vi "Node - Writer.vi"(8 "error in (no error)":errorcluster, 11 "Node Data In":T1) -> (0 "error out":errorcluster, 3 "Node Data Out":T1)   [LabVIEW 2016, in "PXImc Router.lvlib"]
uses:
  PXImc Router.lvlib
  Controls/Node Data.ctl
  <vilib>/NI Veristand/VeriStand Data/Byte Buffer/Byte Buffer.lvclass
  Controls/Node/Node - PXImc Parameters.ctl
  Controls/Node/Transfer Data.ctl
  Controls/Node/Node Ch Properties.ctl
  Controls/Data Type.ctl
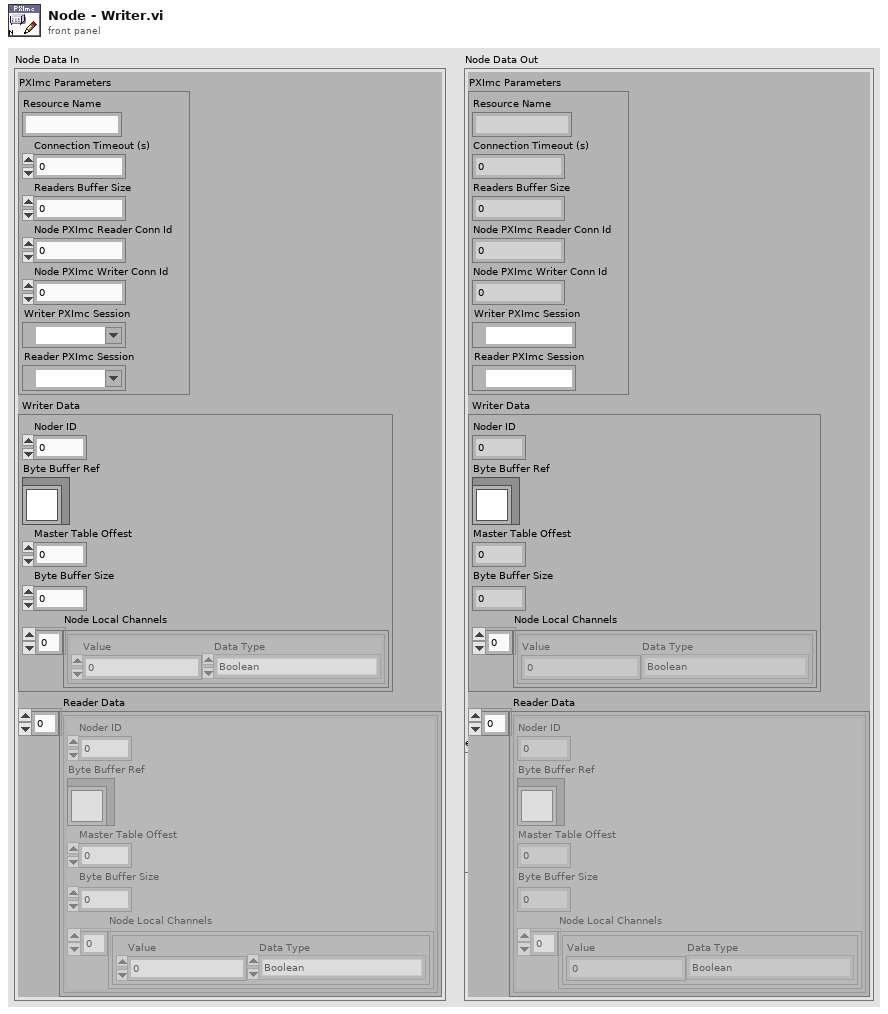
[diagram p1: front panel]
types:
  T1 = typedef "PXImc Router.lvlib/Node Data.ctl" = cluster{"PXImc Parameters":T2, "Writer Data":T3, "Reader Data":T3[]}
  T2 = typedef "PXImc Router.lvlib/Node - PXImc Parameters.ctl" = cluster{"Resource Name":string, "Connection Timeout (s)":dbl, "Readers Buffer Size":u32, "Node PXImc Reader Conn Id":u16, "Node PXImc Writer Conn Id":u16, "Writer PXImc Session":refnum<k21>, "Reader PXImc Session":refnum<k21>}
  T3 = typedef "PXImc Router.lvlib/Transfer Data.ctl" = cluster{"Noder ID":u32, "Byte Buffer Ref":refnum<class "Byte Buffer.lvclass">, "Master Table Offest":u32, "Byte Buffer Size":u32, "Node Local Channels":T4[]}
  T4 = typedef "PXImc Router.lvlib/Node Ch Properties.ctl" = cluster{"Value":dbl, "Data Type":T5}
  T5 = typedef "PXImc Router.lvlib/Data Type.ctl" = enum16{"Boolean", "SGL", "DBL", "I8", "I16", "I32", "I64", "U8", "U16", "U32", "U64"}
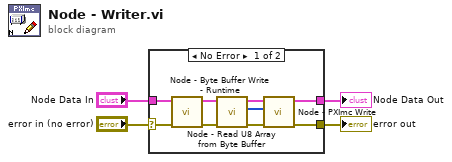
[diagram p0: block diagram]
diagram:
  n1 = case shown="No Error" "error in (no error)" {
    selector: "error in (no error)" -> [w7 w15]
    tunnel: [w13 w15] -> w4
    tunnel: "Node Data In" -> [w8 w14]
    tunnel: [w11 w14] -> w1
    frame No Error {
      n2 = call "Node - Byte Buffer Write - Runtime.vi"("error in (no error)"=w7, "Node Data In"=w8) -> ("error out"=w6:errorcluster, "Node Data Out"=w5:T1)  [unwired: 7 in, 1 out]
      n3 = call "Node - Read U8 Array from Byte Buffer.vi"("error in (no error)"=w6, "Node Data In"=w5) -> ("error out"=w12:errorcluster, "U8 Array Out"=w9:u8[], "Node Data Out"=w10:T1)  [unwired: 7 in]
      n4 = call "Node - PXImc Write.vi"("error in (no error)"=w12, "Writer Data In"=w9, "Node Data In"=w10) -> ("error out"=w13:errorcluster, "Node Data Out"=w11:T1)  [unwired: 7 in]
    }
    frame Error {
    }
  }
  "error out" <- w4
  "Node Data Out" <- w1
